vi "gama2 gama3.vi"(4 "v01^2":dbl[](array[numeric]), 6 "u01^2":dbl[](array[numeric]), 9 "Z":dbl, 10 "v02^2":dbl[](array[numeric]), 11 "u02^2":dbl[](array[numeric])) -> (0 "Bu above":dbl[](array[numeric]), 1 "Au above":dbl[](array[numeric]), 2 "Bp above":dbl[](array[numeric]), 3 "gamma3^2":dbl[](array[numeric]))   [LabVIEW 2021]
panel:
  in  "dV":dbl=0.0001
  out "Waveform Graph":cluster{dbl, "dV":dbl, dbl[][]}(graph)
  out "gamma2^2":dbl[](array[numeric])
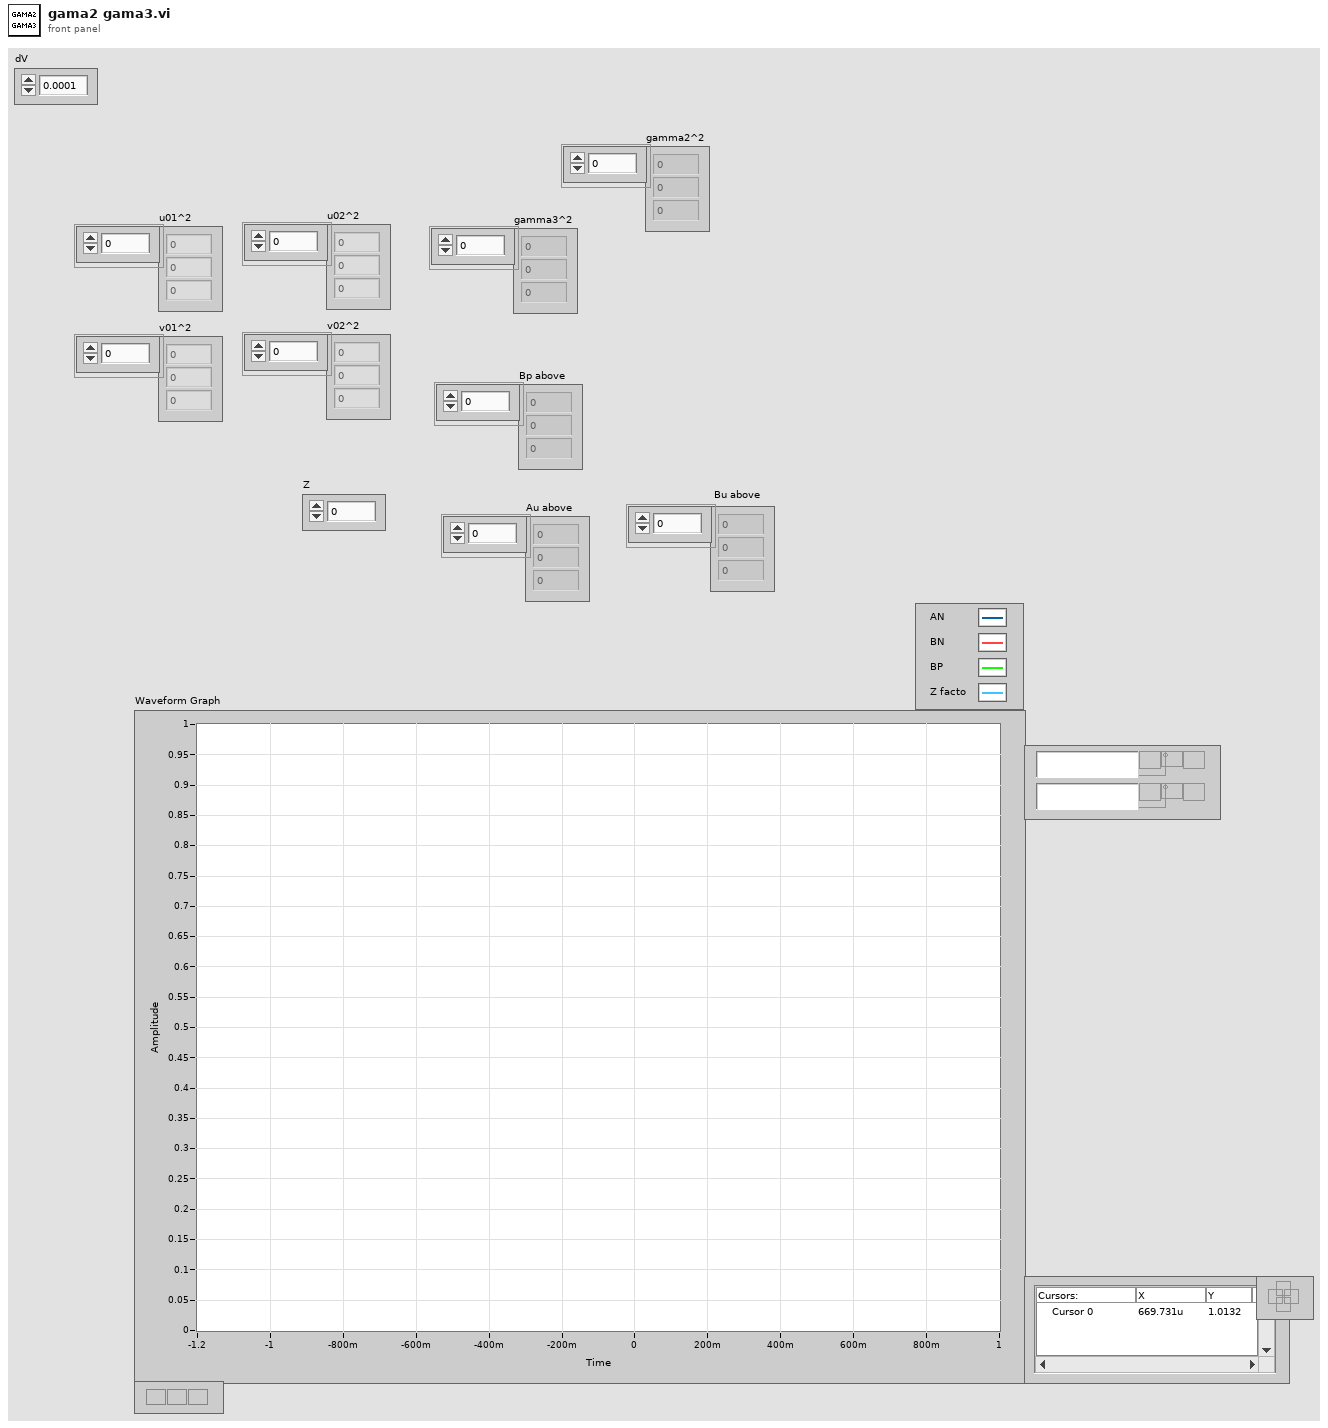
[diagram p1: front panel]
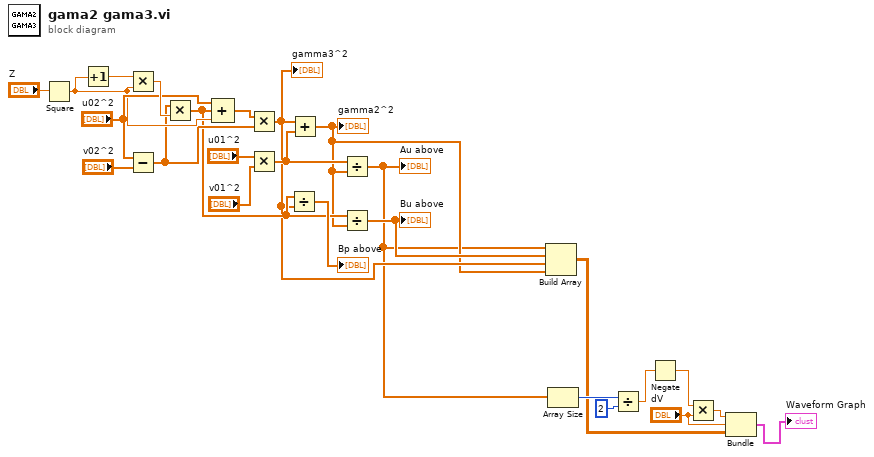
[diagram p0: block diagram]
diagram:
  n1 = Square(x="Z") -> (x^2=w20:dbl)
  n2 = Increment(x=w20) -> (x+1=w23:dbl)
  n3 = Multiply(x=w23, y=w20) -> (x*y=w22:dbl)
  n4 = Subtract(x="u02^2", y="v02^2") -> (x-y=w18:dbl[])
  n5 = Multiply(x=w18, y=w22) -> (x*y=w13:dbl[])
  n6 = Compound Arithmetic op=ADD("u02^2", w13, w20) -> (w19:dbl[])
  n7 = Multiply(x=w19, y=w18) -> (x*y=w5:dbl[])
  "gamma3^2" <- w5
  n8 = Multiply(x="u01^2", y="v01^2") -> (x*y=w14:dbl[])
  n9 = Divide(x=w13, y=w5) -> (x/y=→"Bp above":dbl[])
  n10 = Add(x=w5, y=w14) -> (x+y=w4:dbl[])
  "gamma2^2" <- w4
  n11 = Divide(x=w14, y=w4) -> (x/y=w2:dbl[])
  "Au above" <- w2
  n12 = Divide(x=w13, y=w4) -> (x/y=w6:dbl[])
  "Bu above" <- w6
  n13 = Build Array(w2, w6, w5, w4) -> (w3:dbl[][])
  n14 = Array Size(array=w2) -> (size(s)=w12:i32)
  n15 = Divide(x=w12, y=2) -> (x/y=w10:dbl)
  n16 = Negate(x=w10) -> (-x=w9:dbl)
  n17 = Multiply(x=w9, y="dV") -> (x*y=w8:dbl)
  n18 = Bundle(w8, "dV"="dV", w3) -> (→"Waveform Graph":cluster{dbl, "dV":dbl, dbl[][]})  [unwired: 1 in]
